vi "Read Response.vi"(8 "error in (no error)":errorcluster, 11 "VisaComms in":refnum<class "VisaComms.lvclass">) -> (0 "error out":errorcluster, 2 "Response":string, 3 "VisaComms out":refnum<class "VisaComms.lvclass">, 5 "Buffer":string)   [LabVIEW 2020, in "CTI.lvlib" / "VisaComms.lvclass"]
uses:
  VisaComms.lvclass
  VisaComms.lvclass/VisaComms.ctl
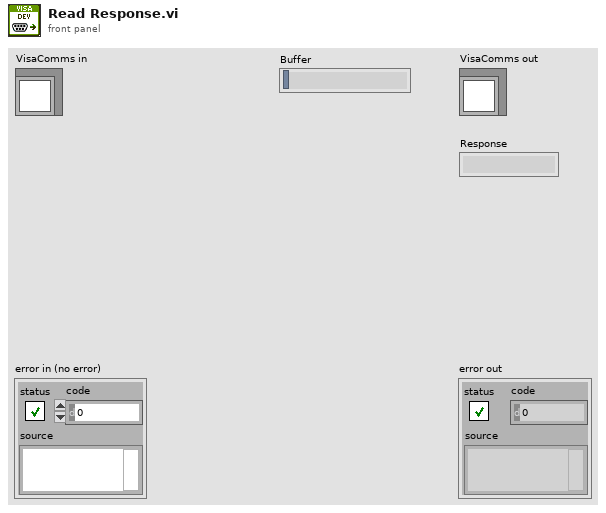
[diagram p1: front panel]
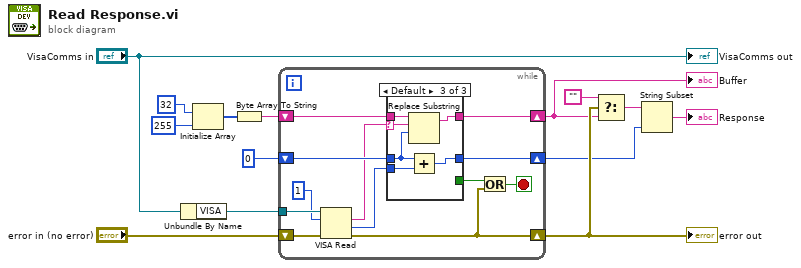
[diagram p0: block diagram]
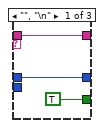
[diagram p2: hidden frame]
diagram:
  n1 = Unbundle By Name("VisaComms in") -> ("VISA"=w4:refnum<visa-resource-name>)
  n2 = Initialize Array(u8 32 ("element"), 255 ("dimension size")) -> (w11:u8[])
  n3 = Byte Array To String(unsigned byte array=w11) -> (string=w7:string)
  n4 = while {
    shift-right: [w17] -> w14
    shift-left: "error in (no error)" -> [w25]
    shift-right: [w20] -> w1
    shift-left: w7 -> [w23]
    shift-right: [w21] -> w8
    shift-left: u32 0 -> [w22]
    tunnel: w4 -> [w26]
    stop <- w18 stop-if-true
    n5 = VISA Read(VISA resource name=w26, byte count=u32 1, error in (no error)=w25) -> (read buffer=w16:string, return count=w19:u32, error out=w17:errorcluster)  [unwired: 1 out]
    n6 = case shown="Default" w16 {
      selector: w16 -> [_ _ w32]
      tunnel: w23 -> [w29 w31 w37]
      tunnel: w22 -> [w28 w30 w36]
      tunnel: [w28 w30 w35] -> w21
      tunnel: [w29 w31 w34] -> w20
      tunnel: w19 -> [_ _ w33]
      tunnel: [TRUE _ _] -> w15
      frame "", "\n" {
      }
      frame "\r" {
      }
      frame Default {
        n7 = Replace Substring(3:w36, 4:w32, 5:w37) -> (1:w34:string)  [unwired: 1 in, 1 out]
        n8 = Add(x=w36, y=w33) -> (x+y=w35:u32)
      }
    }
    n9 = Or(x=w15, y=w17) -> (x .or. y?=w18:bool)
  }
  "error out" <- w14
  "Buffer" <- w1
  n10 = Select(t="", s=w14, f=w1) -> (s? t:f=w9:string)
  n11 = String Subset(string=w9, length (rest)=w8) -> (substring=→"Response":string)  [unwired: 1 in]
  "VisaComms out" <- "VisaComms in"
